vi "Arm.vi"(10 "Down?":bool, 11 "Enum":enum16{"Init", "Run", "End"}(ring)) -> ()   [LabVIEW 2011]
uses:
  TypeDefs/PWM Module 1.ctl
  <vilib>/Rock Robotics/SystemInterfaces/Typedef/FPGA_TypedefDigitalModule.ctl
  <vilib>/Rock Robotics/SystemInterfaces/DIO/FPGA_DIOPWMChannel.ctl
  <vilib>/Rock Robotics/SystemInterfaces/DIO/FPGA_DIORelayChannel.ctl
  <vilib>/Rock Robotics/WPI/MotorControl/WPI_MotorControlOpen Victor.vi
panel:
  in  "PWM Module (DIO A)":T1={"Module"=enum."Digital Module 1", "Shooter Wheel"=enum."PWM 1", "Unassigned"=enum."PWM 2", "Unassigned"=enum."PWM 3", "Unassigned"=enum."PWM 4", "Unassigned"=enum."PWM 5", "Arm Servo"=enum."PWM 6", "Arm"=enum."PWM 7", "Ball Intake"=enum."PWM 8", "Conveyor Belt"=enum."PWM 9", "Shooter Feeder"=enum."PWM 10", "Camera Light"=enum."Relay 1", "Unassigned"=enum."Relay 2", "Unassigned"=enum."Relay 3", "Unassigned"=enum."Relay 4", "Unassigned"=enum."Relay 5", "Unassigned"=enum."Relay 6", "Unassigned"=enum."Relay 7", "Unassigned "=enum."Relay 8"}
  in  "Down":dbl=-0.65
  in  "Up":dbl=0.6
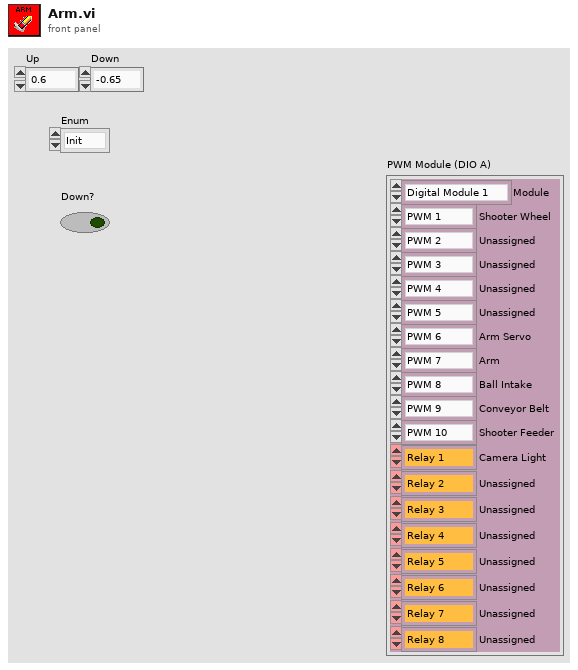
[diagram p1: front panel]
types:
  T1 = typedef "PWM Module 1.ctl" = cluster{"Module":T2, "Shooter Wheel":T3, "Unassigned":T3, "Unassigned":T3, "Unassigned":T3, "Unassigned":T3, "Arm Servo":T3, "Arm":T3, "Ball Intake":T3, "Conveyor Belt":T3, "Shooter Feeder":T3, "Camera Light":T4, "Unassigned":T4, "Unassigned":T4, "Unassigned":T4, "Unassigned":T4, "Unassigned":T4, "Unassigned":T4, "Unassigned ":T4}
  T2 = typedef "FPGA_TypedefDigitalModule.ctl" = enum16{"Digital Module 1", "Digital Module 2"}
  T3 = typedef "FPGA_DIOPWMChannel.ctl" = enum8{"PWM 1", "PWM 2", "PWM 3", "PWM 4", "PWM 5", "PWM 6", "PWM 7", "PWM 8", "PWM 9", "PWM 10", "Invalid"}
  T4 = typedef "FPGA_DIORelayChannel.ctl" = enum8{"Relay 1", "Relay 2", "Relay 3", "Relay 4", "Relay 5", "Relay 6", "Relay 7", "Relay 8", "Invalid"}
  T5 = typedef "WPI_MotorControlDeviceRef.ctl" = cluster{"DeviceStatus":errorcluster, "Type":enum16{"PWM", "CAN"}, "PWM":cluster{"Digital Module":T2, "PWM Channel":T3, "DeadBand":T6}, "CAN":cluster{"Device Number":u8, "Control Mode":T7, "Semaphore":T8, "Max Vout":dbl}, "Invert":bool, "TransformRef":T9, "InvTransformRef":T9}
  T6 = typedef "WPI_PWMDeadband.ctl" = cluster{"Name":string, "maxPositivePwm":i32, "minPositivePwm":i32, "centerPwm":i32, "maxNegativePwm":i32, "minNegativePwm":i32, "angularRange":u16}
  T7 = typedef "WPI_CANJaguar_ControlMode.ctl" = enum8{"Percent VBus", "Current", "Speed", "Position", "Voltage"}
  T8 = typedef "Semaphore RefNum" = refnum<k1>
  T9 = typedef "WPI_PWMTransform_ConPane.ctl" = refnum<vi>
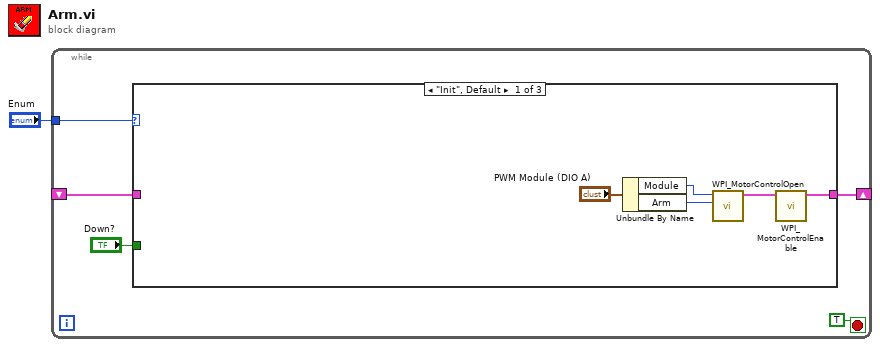
[diagram p0: block diagram]
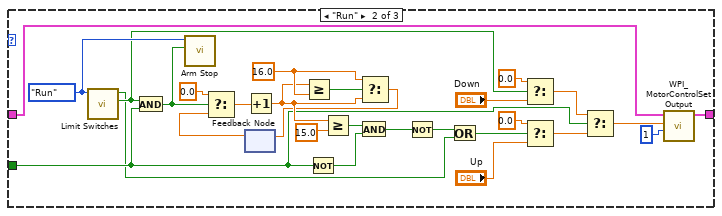
[diagram p2: hidden frame]
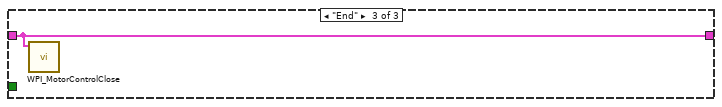
[diagram p3: hidden frame]
diagram:
  n1 = while {
    shift-right: [w5] -> _
    shift-left: _ -> [w6]
    tunnel: "Enum" -> [w3]
    stop <- TRUE stop-if-true
    n2 = case shown="\"Init\", Default" w3 {
      tunnel: w6 -> [_ w39 w40]
      tunnel: [w10 w38 w40] -> w5
      tunnel: "Down?" -> [_ w16 _]
      frame "Init", Default {
        n3 = Unbundle By Name("PWM Module (DIO A)") -> ("Module"=w8:T2, "Arm"=w7:T3)
        n4 = call-poly <vilib>:"WPI_MotorControlOpen.vi"("PWM Channel"=w7, "Digital Module (Module 1)"=w8) -> ("MotorControlDeviceRef"=w11:T5)  [unwired: 8 in, 1 out]
        n5 = call <vilib>:"WPI_MotorControlEnable.vi"("CAN Jaguar Ref"=w11) -> ("CAN Jaguar Ref Out"=w10:T5)  [unwired: 9 in, 1 out]
      }
      frame "Run" {
        w20 = 16.0 ("y")
        w29 = enum16{"Init", "Run", "End"}."Run" ("Enum")
        n6 = call "Limit Switches.vi"("Enum"=w29) -> ("Lower Limit Switch"=w28:bool, "Upper Limit Switch"=w13:bool)  [unwired: 9 in]
        n7 = And(x=w28, y=w16) -> (x .and. y?=w15:bool)
        n8 = call "Arm Stop.vi"("Enum"=w29, "Stop Arm"=w15) -> ()  [unwired: 9 in]
        n9 = feedback #1() -> (w25:dbl)  [unwired: 1 in]
        n10 = Select(t=0.0, s=w15, f=w25) -> (s? t:f=w26:dbl)
        n11 = Increment(x=w26) -> (x+1=w19:dbl)
        n12 = Greater Or Equal?(x=w19, y=w20) -> (x >= y?=w21:bool)
        n13 = Not(x=w16) -> (.not. x?=w22:bool)
        n14 = Greater Or Equal?(x=w19, y=15.0) -> (x >= y?=w23:bool)
        n15 = And(x=w23, y=w22) -> (x .and. y?=w17:bool)
        n16 = Select(t=w20, s=w21, f=w19) -> (s? t:f=w18:dbl)
        n17 = feedback-in #1(w18) -> ()
        n18 = Not(x=w17) -> (.not. x?=w14:bool)
        n19 = Or(x=w14, y=w13) -> (x .or. y?=w12:bool)
        n20 = Select(t=0.0, s=w28, f="Down") -> (s? t:f=w35:dbl)
        n21 = Select(t=0.0, s=w12, f="Up") -> (s? t:f=w36:dbl)
        n22 = Select(t=w35, s=w16, f=w36) -> (s? t:f=w32:dbl)
        n23 = call <vilib>:"WPI_MotorControlSetOutput.vi"("Sync Group"=u8 1, "Output"=w32, "MotorControlDevRef"=w39) -> ("MotorControlDevRef"=w38:T5)  [unwired: 7 in, 1 out]
      }
      frame "End" {
        n24 = call <vilib>:"WPI_MotorControlClose.vi"("MotorControlDevRef"=w40) -> ()  [unwired: 10 in, 1 out]
      }
    }
  }
